vi "WRITE VI.vi"() -> ()   [LabVIEW 2016]
panel:
  in  "BATTERY MEASUREMENTS":bool
  in  "VISA Refnum in":refnum<visa-resource-name>
  in  "error in (no error)":errorcluster
  in  "Numeric":i32
  out "VISA Refnum out":refnum<visa-resource-name>
  out "error out":errorcluster
  out "Bytes at Port":u32
  in  "COUNT":u32
  out "string":string
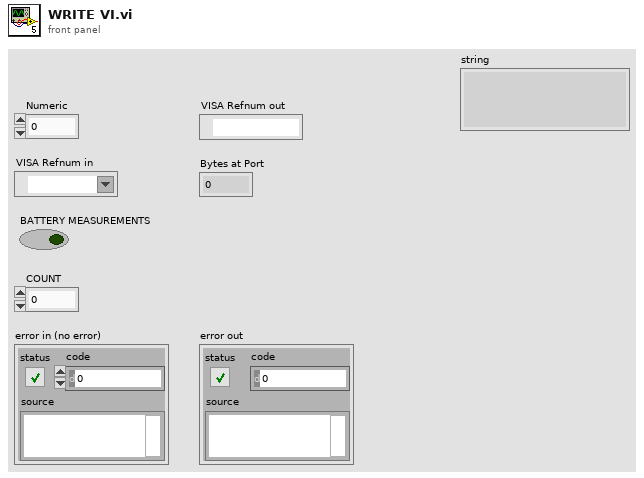
[diagram p1: front panel]
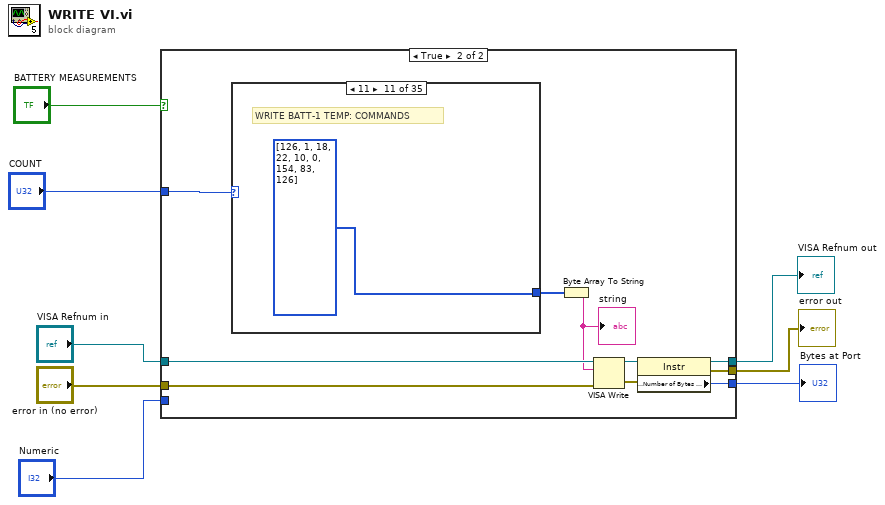
[diagram p0: block diagram]
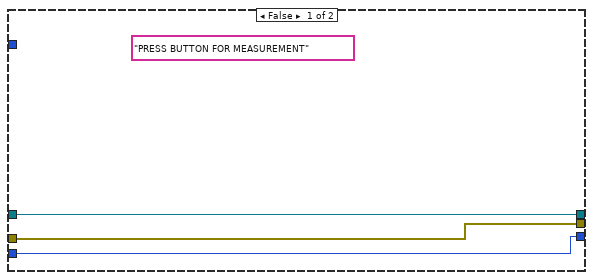
[diagram p2: hidden frame]
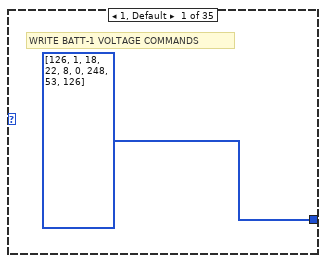
[diagram p3: hidden frame]
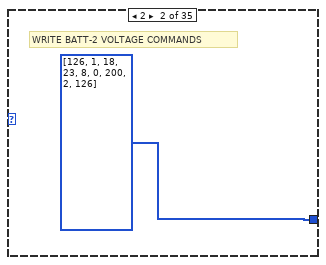
[diagram p4: hidden frame]
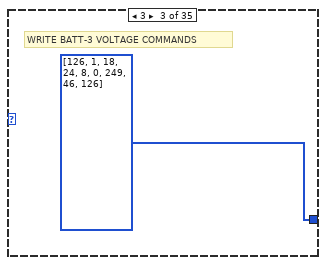
[diagram p5: hidden frame]
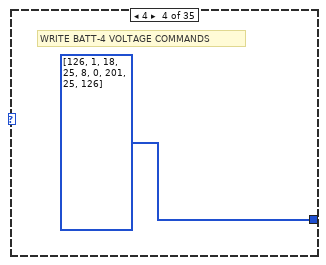
[diagram p6: hidden frame]
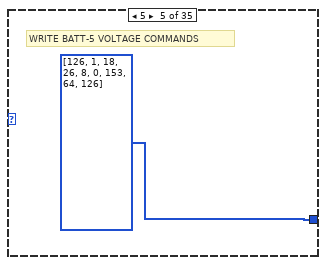
[diagram p7: hidden frame]
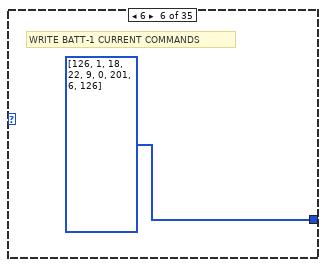
[diagram p8: hidden frame]
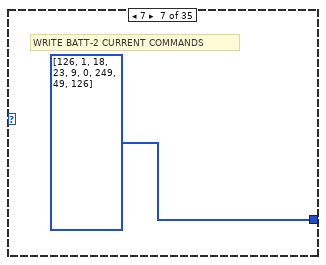
[diagram p9: hidden frame]
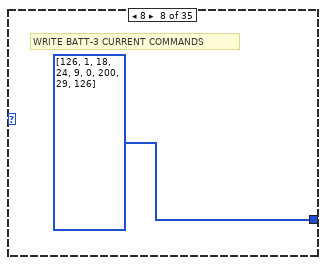
[diagram p10: hidden frame]
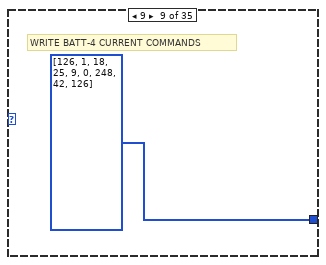
[diagram p11: hidden frame]
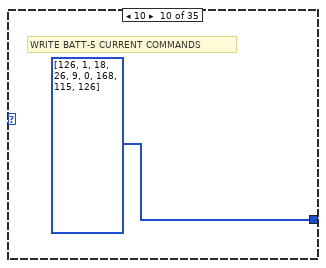
[diagram p12: hidden frame]
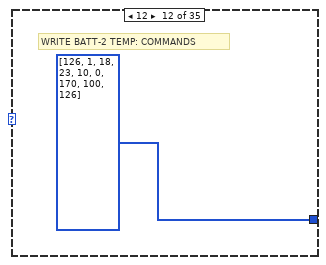
[diagram p13: hidden frame]
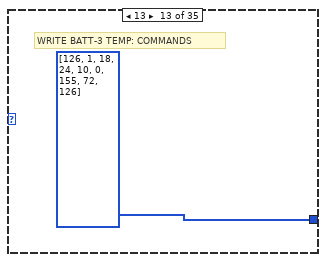
[diagram p14: hidden frame]
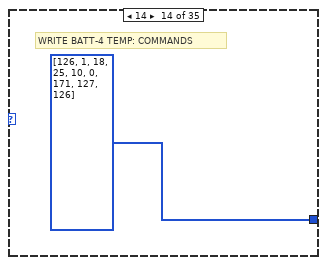
[diagram p15: hidden frame]
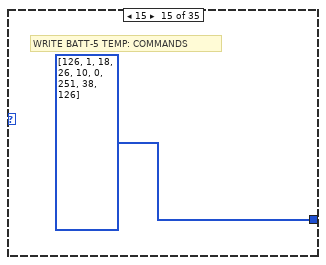
[diagram p16: hidden frame]
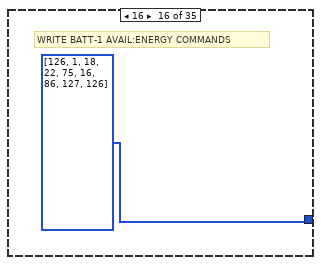
[diagram p17: hidden frame]
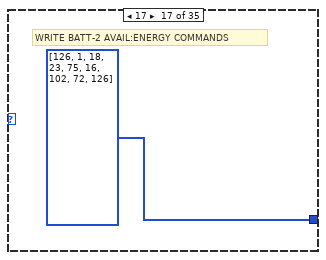
[diagram p18: hidden frame]
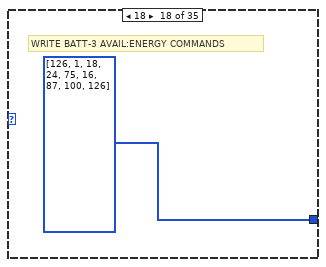
[diagram p19: hidden frame]
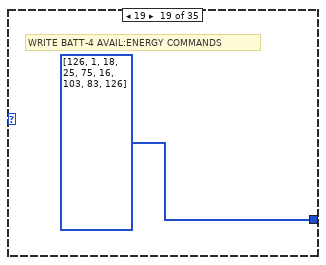
[diagram p20: hidden frame]
diagram:
  n1 = case shown="True" "BATTERY MEASUREMENTS" {
    tunnel: "COUNT" -> [_ w13]
    tunnel: "error in (no error)" -> [w11 w16]
    tunnel: [w9 w19] -> w6
    tunnel: [w11 w18] -> w7
    tunnel: [w10 w17] -> w8
    tunnel: "Numeric" -> [w10 _]
    tunnel: "VISA Refnum in" -> [w9 w15]
    frame False {
      (unwired) "PRESS BUTTON FOR MEASUREMENT"
    }
    frame True {
      n2 = case shown="11" w13 {
        tunnel: [u32[] [126, 1, 18, 22, 8, 0, 248, 53, 126] u32[] [126, 1, 18, 23, 8, 0, 200, 2, 126] u32[] [126, 1, 18, 24, 8, 0, 249, 46, 126] u32[] [126, 1, 18, 25, 8, 0, 201, 25, 126] u32[] [126, 1, 18, 26, 8, 0, 153, 64, 126] i32[] [126, 1, 18, 22, 9, 0, 201, 6, 126] i32[] [126, 1, 18, 23, 9, 0, 249, 49, 126] i32[] [126, 1, 18, 24, 9, 0, 200, 29, 126] i32[] [126, 1, 18, 25, 9, 0, 248, 42, 126] i32[] [126, 1, 18, 26, 9, 0, 168, 115, 126] i16[] [126, 1, 18, 22, 10, 0, 154, 83, 126] i16[] [126, 1, 18, 23, 10, 0, 170, 100, 126] i16[] [126, 1, 18, 24, 10, 0, 155, 72, 126] i16[] [126, 1, 18, 25, 10, 0, 171, 127, 126] i16[] [126, 1, 18, 26, 10, 0, 251, 38, 126] u32[] [126, 1, 18, 22, 75, 16, 86, 127, 126] u32[] [126, 1, 18, 23, 75, 16, 102, 72, 126] u32[] [126, 1, 18, 24, 75, 16, 87, 100, 126] u32[] [126, 1, 18, 25, 75, 16, 103, 83, 126] u32[] [126, 1, 18, 26, 75, 16, 55, 10, 126] u32[] [126, 1, 18, 22, 76, 16, 193, 230, 126] u32[] [126, 1, 18, 23, 76, 16, 241, 209, 126] u32[] [126, 1, 18, 24, 76, 16, 192, 253, 126] u32[] [126, 1, 18, 25, 76, 16, 240, 202, 126] u32[] [126, 1, 18, 26, 76, 16, 160, 147, 126] u32[] [126, 1, 18, 22, 3, 17, 18, 235, 126] u32[] [126, 1, 18, 23, 3, 17, 34, 220, 126] u32[] [126, 1, 18, 24, 3, 17, 19, 240, 126] u32[] [126, 1, 18, 25, 3, 17, 35, 199, 126] u32[] [126, 1, 18, 26, 3, 17, 115, 158, 126] u32[] [126, 1, 18, 22, 4, 17, 133, 114, 126] u32[] [126, 1, 18, 23, 4, 17, 181, 69, 126] u32[] [126, 1, 18, 24, 4, 17, 132, 105, 126] u32[] [126, 1, 18, 25, 4, 17, 180, 94, 126] u32[] [126, 1, 18, 26, 4, 17, 228, 7, 126]] -> w14
        frame 1, Default {
          # "WRITE BATT-1 VOLTAGE COMMANDS"
        }
        frame 2 {
          # "WRITE BATT-2 VOLTAGE COMMANDS"
        }
        frame 3 {
          # "WRITE BATT-3 VOLTAGE COMMANDS"
        }
        frame 4 {
          # "WRITE BATT-4 VOLTAGE COMMANDS"
        }
        frame 5 {
          # "WRITE BATT-5 VOLTAGE COMMANDS"
        }
        frame 6 {
          # "WRITE BATT-1 CURRENT COMMANDS"
        }
        frame 7 {
          # "WRITE BATT-2 CURRENT COMMANDS"
        }
        frame 8 {
          # "WRITE BATT-3 CURRENT COMMANDS"
        }
        frame 9 {
          # "WRITE BATT-4 CURRENT COMMANDS"
        }
        frame 10 {
          # "WRITE BATT-5 CURRENT COMMANDS"
        }
        frame 11 {
          # "WRITE BATT-1 TEMP: COMMANDS"
        }
        frame 12 {
          # "WRITE BATT-2 TEMP: COMMANDS"
        }
        frame 13 {
          # "WRITE BATT-3 TEMP: COMMANDS"
        }
        frame 14 {
          # "WRITE BATT-4 TEMP: COMMANDS"
        }
        frame 15 {
          # "WRITE BATT-5 TEMP: COMMANDS"
        }
        frame 16 {
          # "WRITE BATT-1 AVAIL:ENERGY COMMANDS"
        }
        frame 17 {
          # "WRITE BATT-2 AVAIL:ENERGY COMMANDS"
        }
        frame 18 {
          # "WRITE BATT-3 AVAIL:ENERGY COMMANDS"
        }
        frame 19 {
          # "WRITE BATT-4 AVAIL:ENERGY COMMANDS"
        }
        frame 20 {
          # "WRITE BATT-5 AVAIL:ENERGY COMMANDS"
        }
        frame 21 {
          # "WRITE BATT-1 MAX:ENERGY COMMANDS"
        }
        frame 22 {
          # "WRITE BATT-2 MAX:ENERGY COMMANDS"
        }
        frame 23 {
          # "WRITE BATT-3 MAX:ENERGY COMMANDS"
        }
        frame 24 {
          # "WRITE BATT-4 MAX:ENERGY COMMANDS"
        }
        frame 25 {
          # "WRITE BATT-5 MAX:ENERGY COMMANDS"
        }
        frame 26 {
          # "WRITE BATT-1 REM: CAPACITY COMMANDS"
        }
        frame 27 {
          # "WRITE BATT-2 REM: CAPACITY COMMANDS"
        }
        frame 28 {
          # "WRITE BATT-3 REM: CAPACITY COMMANDS"
        }
        frame 29 {
          # "WRITE BATT-4 REM: CAPACITY COMMANDS"
        }
        frame 30 {
          # "WRITE BATT-5 REM: CAPACITY COMMANDS"
        }
        frame 31 {
          # "WRITE BATT-1 FULL: CAPACITY COMMANDS"
        }
        frame 32 {
          # "WRITE BATT-2 FULL: CAPACITY COMMANDS"
        }
        frame 33 {
          # "WRITE BATT-3 FULL: CAPACITY COMMANDS"
        }
        frame 34 {
          # "WRITE BATT-4 FULL: CAPACITY COMMANDS"
        }
        frame 35 {
          # "WRITE BATT-5 FULL: CAPACITY COMMANDS"
        }
      }
      n3 = Byte Array To String(unsigned byte array=w14) -> (string=w12:string)
      "string" <- w12
      n4 = VISA Write(VISA resource name=w15, write buffer=w12, error in (no error)=w16) -> (VISA resource name out=w21:refnum<visa-resource-name>, error out=w20:errorcluster)  [unwired: 1 out]
      n5 = property class="Instr"(reference=w21, error in=w20) -> (reference out=w19:refnum<visa-resource-name>, error out=w18:errorcluster, "Serial Settings:Number of Bytes at Serial Port"=w17:u32)
    }
  }
  "Bytes at Port" <- w8
  "error out" <- w7
  "VISA Refnum out" <- w6
